vi "2022.12.3—灰度直方图.vi"() -> ()   [LabVIEW 2018]
uses:
  <vilib>/vision/NI_Vision_Development_Module.lvlib
panel:
  out "波形图":T1(graph)
  out "Image":T2(plugin-control)
  out "Standard  Deviation":sgl format="%.2f"
  out "Mean Value":sgl format="%.2f"
  out "Histogram Graph":T1 {"Incremental Value" format="%.2f"; "Starting Value" format="%.2f"}
  in  "停止":bool
  in  "File Path":path
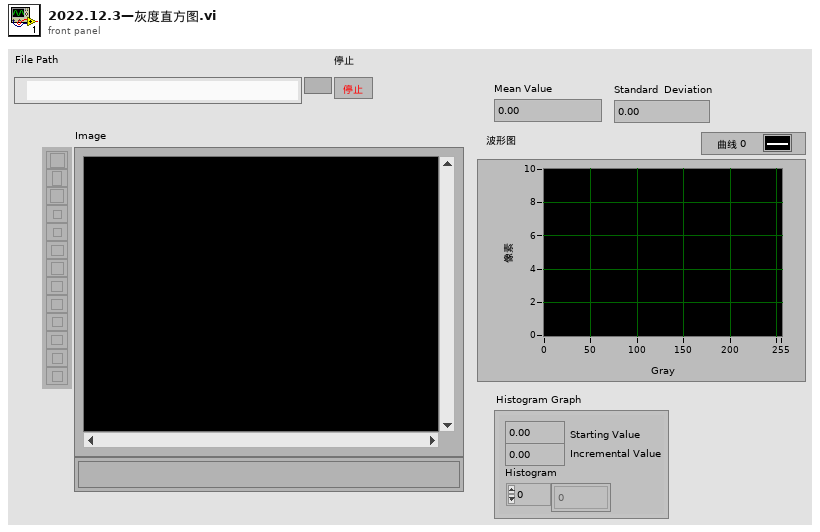
[diagram p1: front panel]
types:
  T1 = cluster{"Starting Value":sgl, "Incremental Value":sgl, "Histogram":u32[]}
  T2 = typedef "IMAQ Image.ctl" = refnum<image>
  T3 = typedef "Image Type" = u32
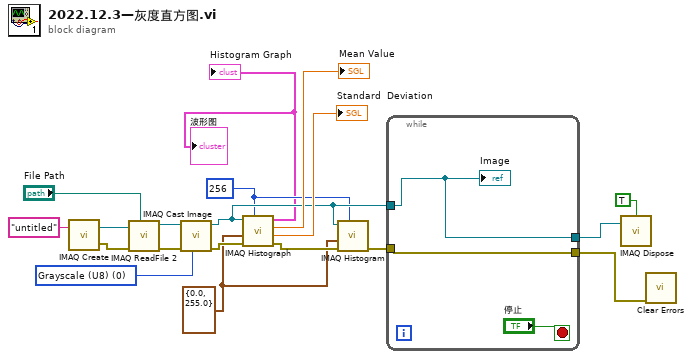
[diagram p0: block diagram]
diagram:
  w4 = cluster{"Minimum":sgl, "Maximum":sgl} {"Minimum"=0.0, "Maximum"=255.0} ("Interval Range")
  w2 = 256 ("Number of Classes")
  w13 = T3 0 items=["Grayscale (U8)", "Grayscale (I16)", "Grayscale (SGL)", "Complex (CSG)", "RGB (U32)", "HSL (U32)", "RGB (U64)", "Grayscale (U16)"] ("Image Type")
  n1 = call "IMAQ Create"("Image Name"="untitled") -> ("New Image"=w18:T2, "error out"=w17:errorcluster)  [unwired: 4 in]
  n2 = call "IMAQ ReadFile 2"("File Path"="File Path", "error in (no error)"=w17, "Image"=w18) -> ("error out"=w16:errorcluster, "Image Out"=w15:T2)  [unwired: 4 in, 3 out]
  n3 = call "IMAQ Cast Image"("Image Type"=w13, "error in (no error)"=w16, "Image Src"=w15) -> ("error out"=w9:errorcluster, "Image Dst Out"=w3:T2)  [unwired: 7 in]
  n4 = call "IMAQ Histograph"("Number of Classes"=w2, "error in (no error)"=w9, "Interval Range"=w4, "Image"=w3) -> ("error out"=w8:errorcluster, "Standard  Deviation"=→"Standard  Deviation":sgl, "Mean Value"=→"Mean Value":sgl, "Histogram Graph"=→"Histogram Graph" →"波形图":T1)  [unwired: 4 in]
  n5 = call "IMAQ Histogram"("Number of Classes"=w2, "error in (no error)"=w8, "Interval Range"=w4, "Image"=w3) -> ("error out"=w5:errorcluster)  [unwired: 6 in, 1 out]
  n6 = while {
    tunnel: [w21] -> w12
    tunnel: [w20] -> w11
    tunnel: w3 -> [w21]
    tunnel: w5 -> [w20]
    stop <- "停止" stop-if-true
    "Image" <- w21
  }
  n7 = call "IMAQ Dispose"("All Images? (No)"=TRUE, "Image"=w12) -> ()  [unwired: 4 in, 1 out]
  n8 = call <vilib>:"Clear Errors.vi"("error in (no error)"=w11) -> ()  [unwired: 5 in, 2 out]
